vi "registerPublisherReply.vi"(2 "Publisher":T1, 3 "ROS_Master.lvclass in":refnum<class "ROS_Master.lvclass">) -> (0 "XML":string)   [LabVIEW 2013, in "ROS_Master.lvclass"]
uses:
  <userlib>/ROS_Master/ROS_Master.lvclass
  <userlib>/ROS_Master/ROS_Master.lvclass/ROS_Master.ctl
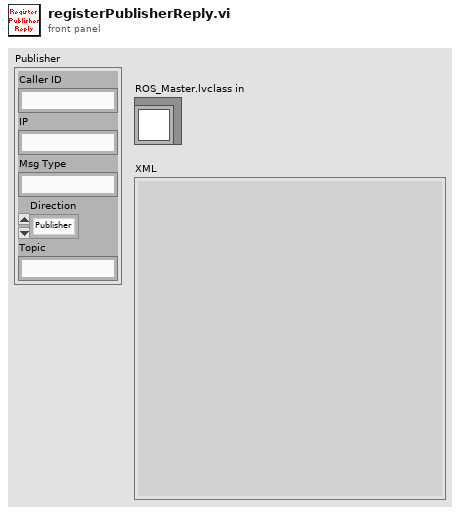
[diagram p1: front panel]
types:
  T1 = cluster{"Caller ID":string, "IP":string, "Msg Type":string, "Direction":enum16{"Publisher", "Subscriber"}, "Topic":string}
  T2 = cluster{"Name":string, "PubSubs":cluster{"Caller ID":string, "IP":string, "Msg Type":string, "Direction":enum16{"Publisher", "Subscriber"}, "Topic":string}[]}[]
  T3 = cluster{"Caller ID":string, "IP":string, "Msg Type":string, "Direction":enum16{"Publisher", "Subscriber"}, "Topic":string}[]
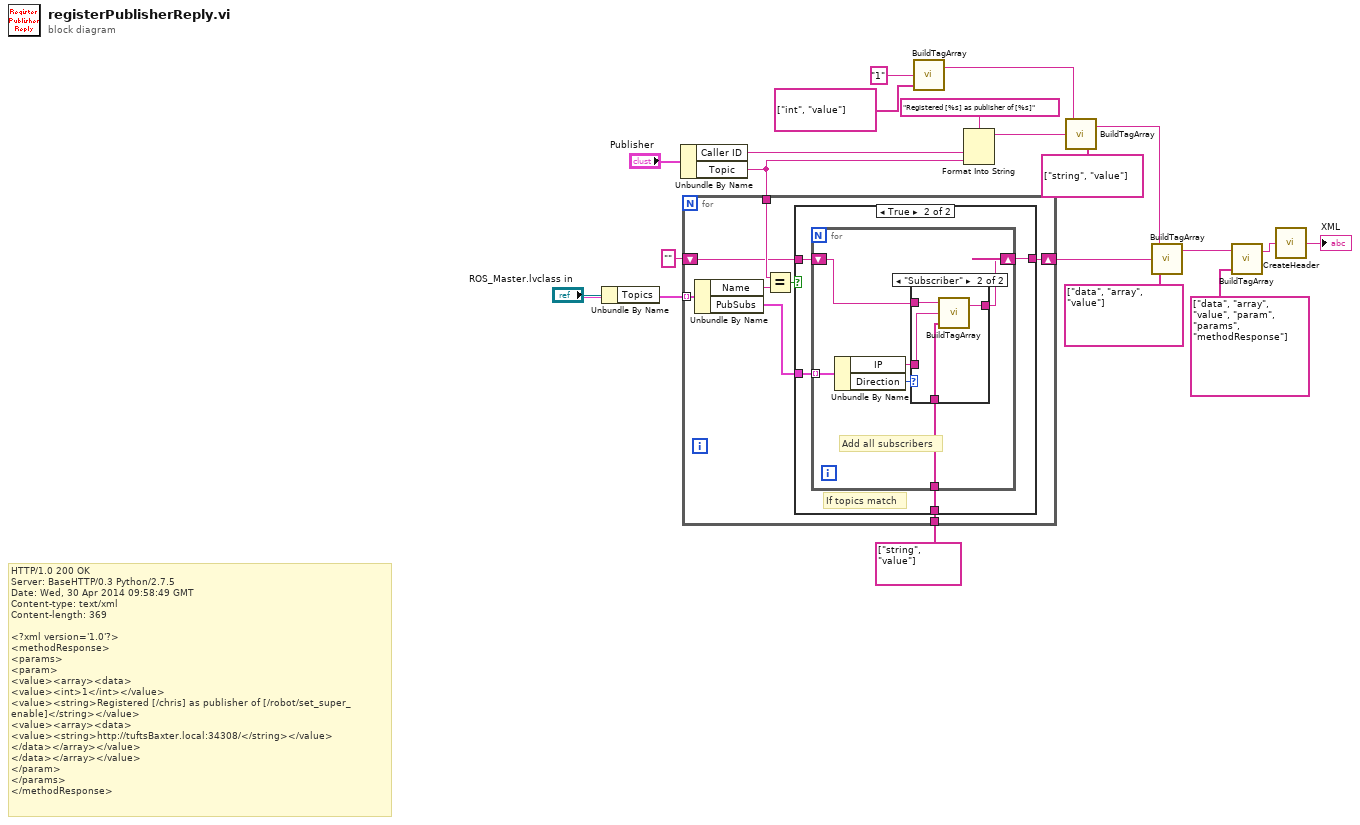
[diagram p0: block diagram]
diagram:
  # "HTTP/1.0 200 OK\nServer: BaseHTTP/0.3 Python/2.7.5\nDate: Wed, 30 Apr 2014 09:58:49 GMT\nContent-type: text/xml\nContent-length: 369\n\n<?xml version='1.0'?>\n<methodResponse>\n<params>\n<param>\n<value><array><data>\n<value><int>1</int></value>\n<value><string>Registered [/chris] as publisher of [/robot/set_super_enable]</string></value>\n<value><array><data>\n<value><string>http://tuftsBaxter.local:34308/</string></value>\n</data></array></value>\n</data></array></value>\n</param>\n</params>\n</methodResponse>"
  n1 = Unbundle By Name("ROS_Master.lvclass in") -> ("Topics"=w19:T2)
  n2 = Unbundle By Name("Publisher") -> ("Caller ID"=w14:string, "Topic"=w2:string)
  n3 = for {
    tunnel: w2 -> [w23]
    tunnel: w19 -> [w28] mode=indexing
    shift-right: [w27] -> w17
    shift-left: "" ("string out") -> [w21]
    tunnel: string[] ["string", "value"] ("tags") -> [w25]
    n4 = Unbundle By Name(w28) -> ("Name"=w22:string, "PubSubs"=w26:T3)
    n5 = Equal?(x=w23, y=w22) -> (x = y?=w24:bool)
    n6 = case shown="True" w24 {
      tunnel: [w29 w33] -> w27
      tunnel: w26 -> [_ w31]
      tunnel: w25 -> [_ w30]
      tunnel: w21 -> [w29 w32]
      frame False {
      }
      frame True {
        # "If topics match"
        n7 = for {
          shift-right: [w39] -> w33
          shift-left: w32 -> [w36]
          tunnel: w31 -> [w38] mode=indexing
          tunnel: w30 -> [w35]
          # "Add all subscribers"
          n8 = Unbundle By Name(w38) -> ("IP"=w34:string, "Direction"=w37:enum16{"Publisher", "Subscriber"})
          n9 = case shown="\"Subscriber\"" w37 {
            tunnel: [w40 w44] -> w39
            tunnel: w36 -> [w40 w43]
            tunnel: w35 -> [_ w42]
            tunnel: w34 -> [_ w41]
            frame "Publisher", Default {
            }
            frame "Subscriber" {
              n10 = call <userlib>:"BuildTagArray.vi"("tags"=w42, "value"=w41, "string in"=w43) -> ("string out"=w44:string)  [unwired: 1 in]
            }
          }
        }
      }
    }
  }
  n11 = call <userlib>:"BuildTagArray.vi"("tags"=string[] ["int", "value"], "value"="1") -> ("string out"=w9:string)  [unwired: 2 in]
  n12 = Format Into String(format string="Registered [%s] as publisher of [%s]", w14, w2) -> (resulting string=w13:string)  [unwired: 2 in, 1 out]
  n13 = call <userlib>:"BuildTagArray.vi"("tags"=string[] ["string", "value"], "value"=w13, "string in"=w9) -> ("string out"=w8:string)  [unwired: 1 in]
  n14 = call <userlib>:"BuildTagArray.vi"("tags"=string[] ["data", "array", "value"], "value"=w17, "string in"=w8) -> ("string out"=w7:string)  [unwired: 1 in]
  n15 = call <userlib>:"BuildTagArray.vi"("tags"=string[] ["data", "array", "value", "param", "params", "methodResponse"], "value"=w7) -> ("string out"=w5:string)  [unwired: 2 in]
  n16 = call <userlib>:"CreateHeader.vi"("Content"=w5) -> ("XML"=→"XML":string)
